vi "Sort Strings.vi"(0 "Strings":string[](array[string])=["Level 1A/Item 1", "Level 1A/Item 2", "Level 1B/Item 1"], 7 "Delimiter":string="/") -> (8 "Menu Items":T1(array[cluster])=[{"Names"=["Item 1", "Level 1A", "Level 1B"], "Tags"=["Level 1A/Level 1A", "Level 1A", "Level 1B"], "Child"=[1, 2, 4]}, {"Names"=[], "Tags"=[], "Child"=[]}, {"Names"=["Item 2"], "Tags"=["Level 1A/Level 1A"], "Child"=[3]}, {"Names"=[], "Tags"=[], "Child"=[]}, {"Names"=["Item 1"], "Tags"=["Level 1B/Level 1B"], "Child"=[5]}, {"Names"=[], "Tags"=[], "Child"=[]}])   [LabVIEW 2020, in "KMultilevel Ring.xctl"]
uses:
  KMultilevel Ring.xctl
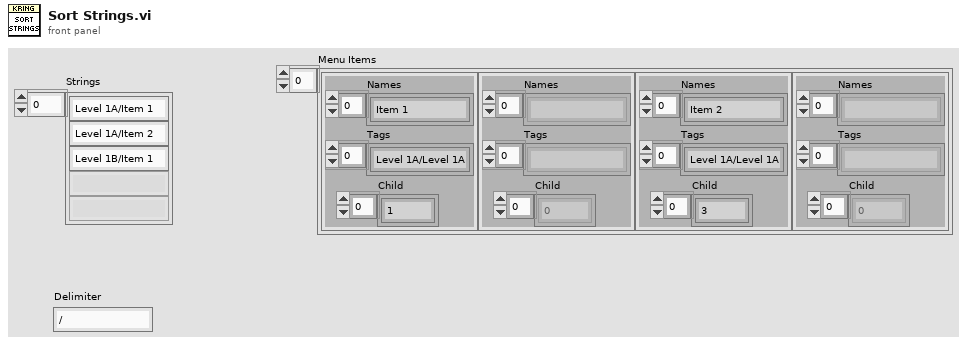
[diagram p1: front panel]
types:
  T1 = cluster{"Names":string[], "Tags":string[], "Child":i32[]}[]
  T2 = cluster{"Names":string[], "Tags":string[], "Child":i32[]}
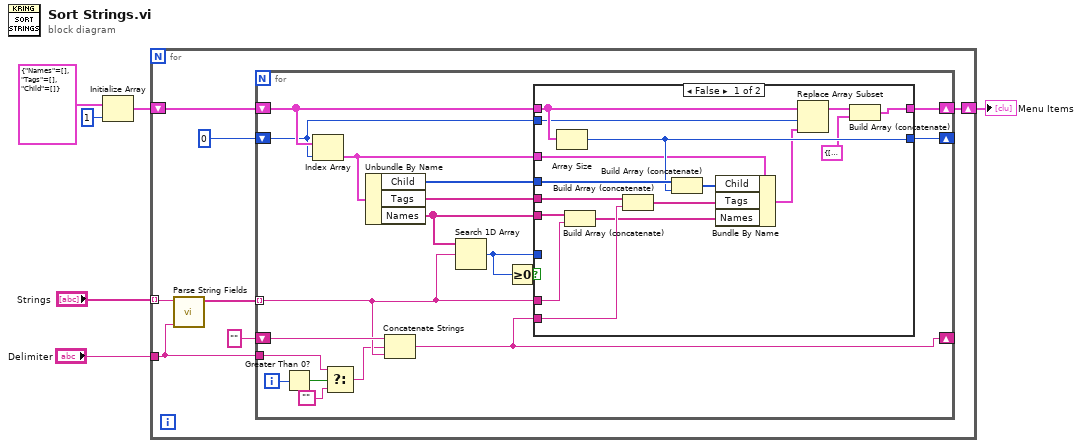
[diagram p0: block diagram]
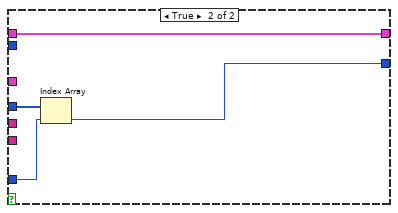
[diagram p2: hidden frame]
diagram:
  n1 = Initialize Array(T2 {"Names"=[], "Tags"=[], "Child"=[]} ("Cluster"), 1 ("dimension size")) -> (w1:T1)
  n2 = for {
    tunnel: "Strings" -> [w13] mode=indexing
    tunnel: "Delimiter" -> [w8]
    shift-right: [w11] -> w4
    shift-left: w1 -> [w12]
    n3 = call "Parse String Fields.vi"("Separator"=w8, "String"=w13) -> ("Fields"=w9:string[])  [unwired: 8 in, 1 out]
    n4 = for {
      tunnel: w9 -> [w24] mode=indexing
      shift-right: [w14] -> _
      shift-left: "" -> [w25]
      shift-right: [w21] -> w11
      shift-left: w12 -> [w22]
      shift-right: [w28] -> _
      shift-left: 0 -> [w20]
      tunnel: w8 -> [w17]
      i -> [w19]
      n5 = Greater Than 0?(x=w19) -> (x > 0?=w18:bool)
      n6 = Index Array(array=w22, index=w20) -> (element=w26:T2)
      n7 = Select(t=w17, s=w18, f="") -> (s? t:f=w16:string)
      n8 = Unbundle By Name(w26) -> ("Child"=w23:i32[], "Tags"=w30:string[], "Names"=w27:string[])
      n9 = Concatenate Strings(w25, w16, w24) -> (w14:string)
      n10 = Search 1D Array(1D array=w27, element=w24) -> (index of element=w29:i32)  [unwired: 1 in]
      n11 = Greater Or Equal To 0?(x=w29) -> (x >= 0?=w31:bool)
      n12 = case shown="False" w31 {
        tunnel: w30 -> [w45 _]
        tunnel: w29 -> [_ w51]
        tunnel: [w42 w50] -> w28
        tunnel: w24 -> [w46 _]
        tunnel: w27 -> [w47 _]
        tunnel: w26 -> [w41 _]
        tunnel: w14 -> [w44 _]
        tunnel: w23 -> [w43 w49]
        tunnel: w22 -> [w37 w48]
        tunnel: w20 -> [w36 _]
        tunnel: [w32 w48] -> w21
        frame False {
          n13 = Array Size(array=w37) -> (size(s)=w42:i32)
          n14 = Build Array (concatenate)(w47, w46) -> (w38:string[])
          n15 = Build Array (concatenate)(w45, w44) -> (w39:string[])
          n16 = Build Array (concatenate)(w43, w42) -> (w40:i32[])
          n17 = Bundle By Name(cluster=w41, "Child"=w40, "Tags"=w39, "Names"=w38) -> (w35:T2)
          n18 = Replace Array Subset(array=w37, new element=w35, index=w36) -> (w34:T1)
          n19 = Build Array (concatenate)(w34, T2 {"Names"=[], "Tags"=[], "Child"=[]} ("Cluster")) -> (w32:T1)
        }
        frame True {
          n20 = Index Array(array=w49, index=w51) -> (element=w50:i32)
        }
      }
    }
  }
  "Menu Items" <- w4
